vi "Load APU Setup.vi"(8 "error in (no error)":errorcluster, 11 "APU Setup File":T1) -> (0 "error out":errorcluster)   [LabVIEW 2018, in "Testing UI 2.lvlib"]
doc: "This subVI enqueues the named action in to the communications queue along with the input data."
uses:
  Testing UI 2.lvlib
  Private Controls/Module Action.ctl
  Top Level/Shared Controls/APU Setup File.ctl
  Private Controls/Module Data.ctl
panel:
  in  "Action":T2=enum."Load APU Setup"
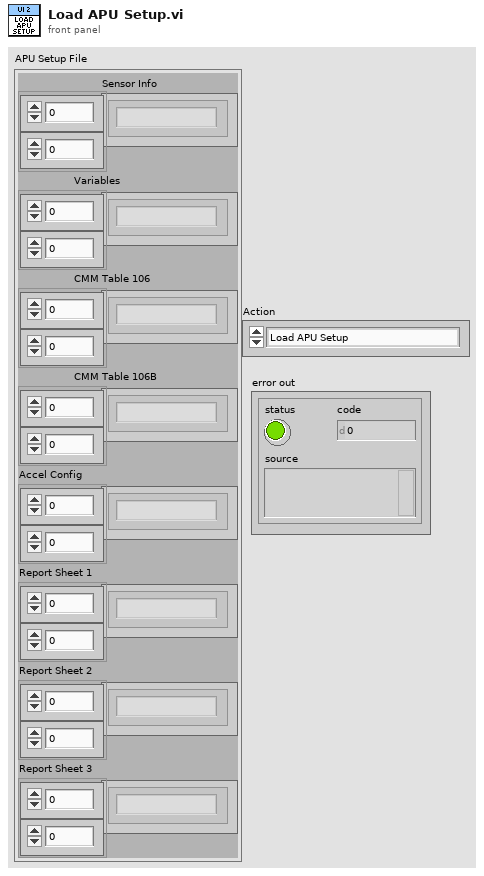
[diagram p1: front panel]
types:
  T1 = typedef "APU Setup File.ctl" = cluster{"Sensor Info":string[][], "Variables":string[][], "CMM Table 106":string[][], "CMM Table 106B ":string[][], "Accel Config":string[][], "Report Sheet 1":string[][], "Report Sheet 2":string[][], "Report Sheet 3":string[][]}
  T2 = typedef "Testing UI 2.lvlib/Module Action.ctl" = enum8{"Init", "Open FP", "Error", "Exit", "Timeout", "Load APU Setup"}
  T3 = typedef "Testing UI 2.lvlib/Module Data.ctl" = cluster{"Data":variant, "Action":T2}
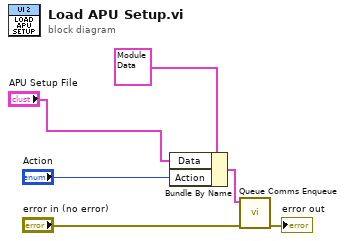
[diagram p0: block diagram]
diagram:
  n1 = Bundle By Name(cluster=T3 {"Data"=variant, "Action"=enum."Init"} ("element"), "Data"="APU Setup File", "Action"="Action") -> (w6:T3)
  n2 = call "Queue Comms Enqueue.vi"("error in (no error)"="error in (no error)", "element"=w6) -> ("error out"=→"error out":errorcluster)  [unwired: 9 in]
